vi "SaveDataFile.vi"(0 "Data Array":dbl[][](array[numeric]), 1 "Temperature":dbl, 2 "Current Sensor":string, 3 "Humidity":dbl, 5 "no. of arrays":i32, 7 "Passed?":bool, 9 "Actual array lengths":i32, 11 "Error In":errorcluster, 12 "Array Titles":string, 13 "Strip Segment":string, 14 "Arrays format":string) -> (4 "Filename OUT":string, 6 "Pathname OUT":string, 10 "Path + Filename OUT":string, 15 "Error Out":errorcluster)   [LabVIEW 2018]
uses:
  globals/QC_RunInformation.vi
  globals/QC_MeasurementSetup.vi
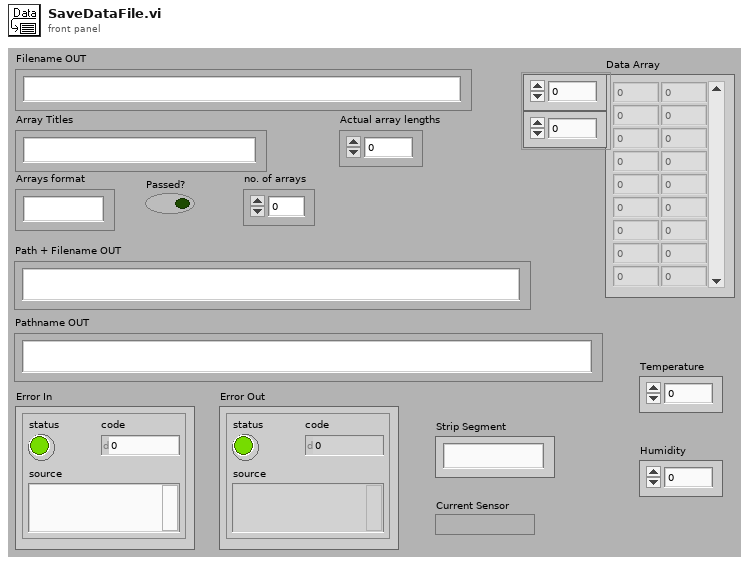
[diagram p1: front panel]
types:
  T1 = enum16{"open", "open or create", "create or replace", "create"}
  T2 = cluster{"Institute":string, "Manufacturers":string[], "Devices":string[], "Serialnumbers Lookup DB":string, "Data directory":string, "Backup & screenshot directory":string, "List of known users":string[]}
  T3 = cluster{"User":string, " Institute":string, " Test Time":string, " Test Date":string, "Instruments":string, "Sensor IDS":string[], "IV Test?":bool, "CV Test? ":bool, "LCS Test? ":bool, "No. of Ch.":u16, " Current Sensor":string, " Current Test":string, "Arduino DP Map":string[], "Sensor BW":string[], "Sensor Types":string[]}
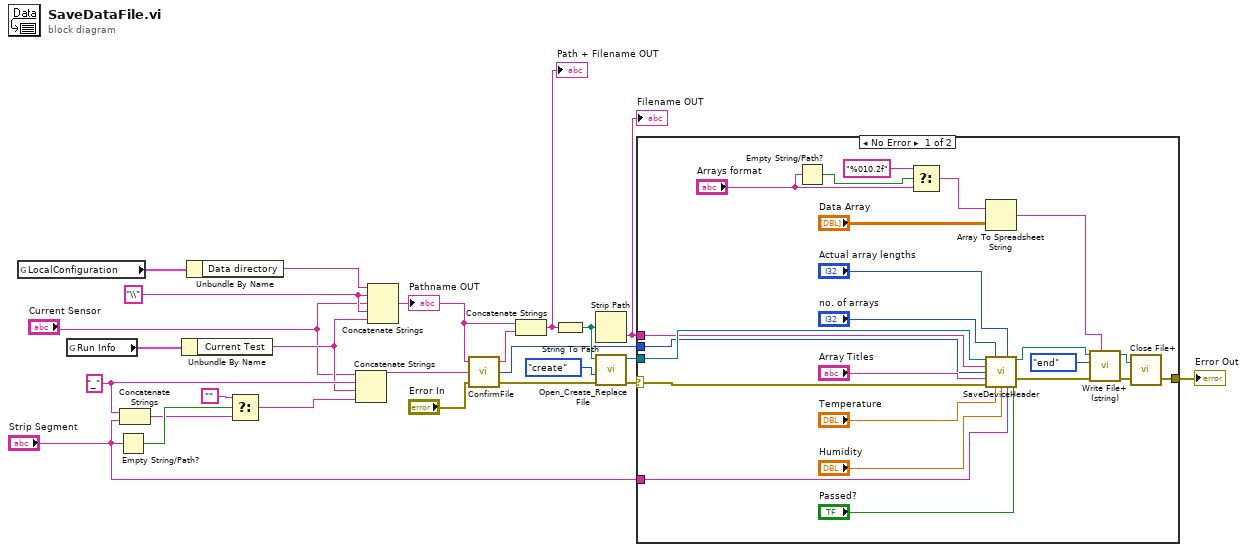
[diagram p0: block diagram]
diagram:
  w8 = "_"
  w18 = "\\"
  n1 = global read "QC_RunInformation.vi" "LocalConfiguration"() -> (w25:T2)
  n2 = global read "QC_MeasurementSetup.vi" "Run Info"() -> (w3:T3)
  n3 = Empty String/Path?(string/path="Strip Segment") -> (empty?=w10:bool)
  n4 = Concatenate Strings(w8, "Strip Segment") -> (w6:string)
  n5 = Unbundle By Name(w3) -> ("Current Test"=w2:string)
  n6 = Unbundle By Name(w25) -> ("Data directory"=w24:string)
  n7 = Select(t="", s=w10, f=w6) -> (s? t:f=w7:string)
  n8 = Concatenate Strings("Current Sensor", w8, w2, w7) -> (w17:string)
  n9 = Concatenate Strings(w24, w18, "Current Sensor", w18, w2) -> (w13:string)
  "Pathname OUT" <- w13
  n10 = call "ConfirmFile.vi"("Error In"="Error In", "Filename IN"=w17, "Pathname IN"=w13) -> ("Error Out"=w14:errorcluster, "Run Number"=w5:i32, "Filename:"=w12:string)
  n11 = Concatenate Strings(w13, w12) -> (w11:string)
  "Path + Filename OUT" <- w11
  n12 = String To Path(string=w11) -> (path=w20:path)
  n13 = Strip Path(path=w20) -> (name=w21:string)  [unwired: 1 out]
  "Filename OUT" <- w21
  n14 = call <vilib>:"Open_Create_Replace File.vi"("error in (no error)"=w14, "function (open:0)"=T1."create", "file path"=w20) -> ("error out"=w19:errorcluster, "refnum"=w22:refnum<file>)  [unwired: 5 in, 2 out]
  n15 = case shown="No Error" w19 {
    selector: w19 -> [w48 w49]
    tunnel: w22 -> [w37 _]
    tunnel: w21 -> [w36 _]
    tunnel: [w32 w49] -> w16
    tunnel: w5 -> [w28 _]
    tunnel: "Strip Segment" -> [w27 _]
    frame No Error {
      n16 = Empty String/Path?(string/path="Arrays format") -> (empty?=w45:bool)
      n17 = Select(t="%010.2f", s=w45, f="Arrays format") -> (s? t:f=w43:string)
      n18 = Array To Spreadsheet String(array="Data Array", 3:w43) -> (spreadsheet string=w42:string)  [unwired: 1 in]
      n19 = call "SaveDeviceHeader.vi"("File Refnum in"=w37, "no. of arrays"="no. of arrays", "Array Lengths"="Actual array lengths", "Filename"=w36, "Run Number"=w28, "Array Titles"="Array Titles", "error in (no error)"=w48, "Temperature"="Temperature", "Humidity"="Humidity", "Strip Segment"=w27, "Passed?"="Passed?") -> ("File Refnum out"=w38:refnum<file>, "error out"=w29:errorcluster)  [unwired: 2 in, 1 out]
      n20 = call <vilib>:"Write File+ (string).vi"("string"=w42, "error in (no error)"=w29, "pos mode (rel. to end:1)"=enum16{"start", "end", "current"}."end", "refnum"=w38) -> ("error out"=w41:errorcluster, "dup refnum"=w39:refnum<file>)  [unwired: 3 in, 1 out]
      n21 = call <vilib>:"Close File+.vi"("error in (no error)"=w41, "refnum"=w39) -> ("error out"=w32:errorcluster)  [unwired: 3 in, 2 out]
    }
    frame Error {
    }
  }
  "Error Out" <- w16
